vi "Page.Next.vi"(8 "error in (no error)":errorcluster, 11 "State Variables":T1) -> (0 "error out":errorcluster, 3 "State Variables":T1)   [LabVIEW 2015]
uses:
  Types/Main.StateVariables.ctl
  <vilib>/Utility/miscctls.llb/LVPositionTypeDef.ctl
  Types/Execute.UserEventRefs.ctl
  <vilib>/NI Veristand/Execution/Workspace/SystemStateRegEventRef.ctl
  <vilib>/NI Veristand/Execution/Workspace/Target State Info.ctl
  <vilib>/NI Veristand/Execution/Workspace/Target State.ctl
  <vilib>/NI Veristand/Execution/WaveformStreaming/Waveform Data Watcher Event Data (DBL).ctl
  <vilib>/NI Veristand/Execution/WaveformStreaming/WaveformStreamSpecification.ctl
  NationalInstruments.VeriStand.ClientAPI
  <vilib>/NI Veristand/Execution/Workspace/SystemStateEventRef.ctl
  <vilib>/NI Veristand/Execution/Workspace/WorkspaceAPI.ctl
  Types/UI.Object.ctl
  Types/Waveforms.Info.ctl
  <vilib>/NI Veristand/Execution/WaveformStreaming/Registered Waveform Streams Data Event Refnum (DBL).ctl
  <vilib>/NI Veristand/Execution/WaveformStreaming/WaveformDataWatcherDBL.ctl
  <vilib>/NI Veristand/Execution/WaveformStreaming/WaveformStreamingAPI.ctl
  <vilib>/NI Veristand/Execution/Workspace/NI_VS Workspace ExecutionAPI.lvlib
  <vilib>/NI Veristand/Execution/WaveformStreaming/NI_VS Waveform Streaming Interface.lvlib
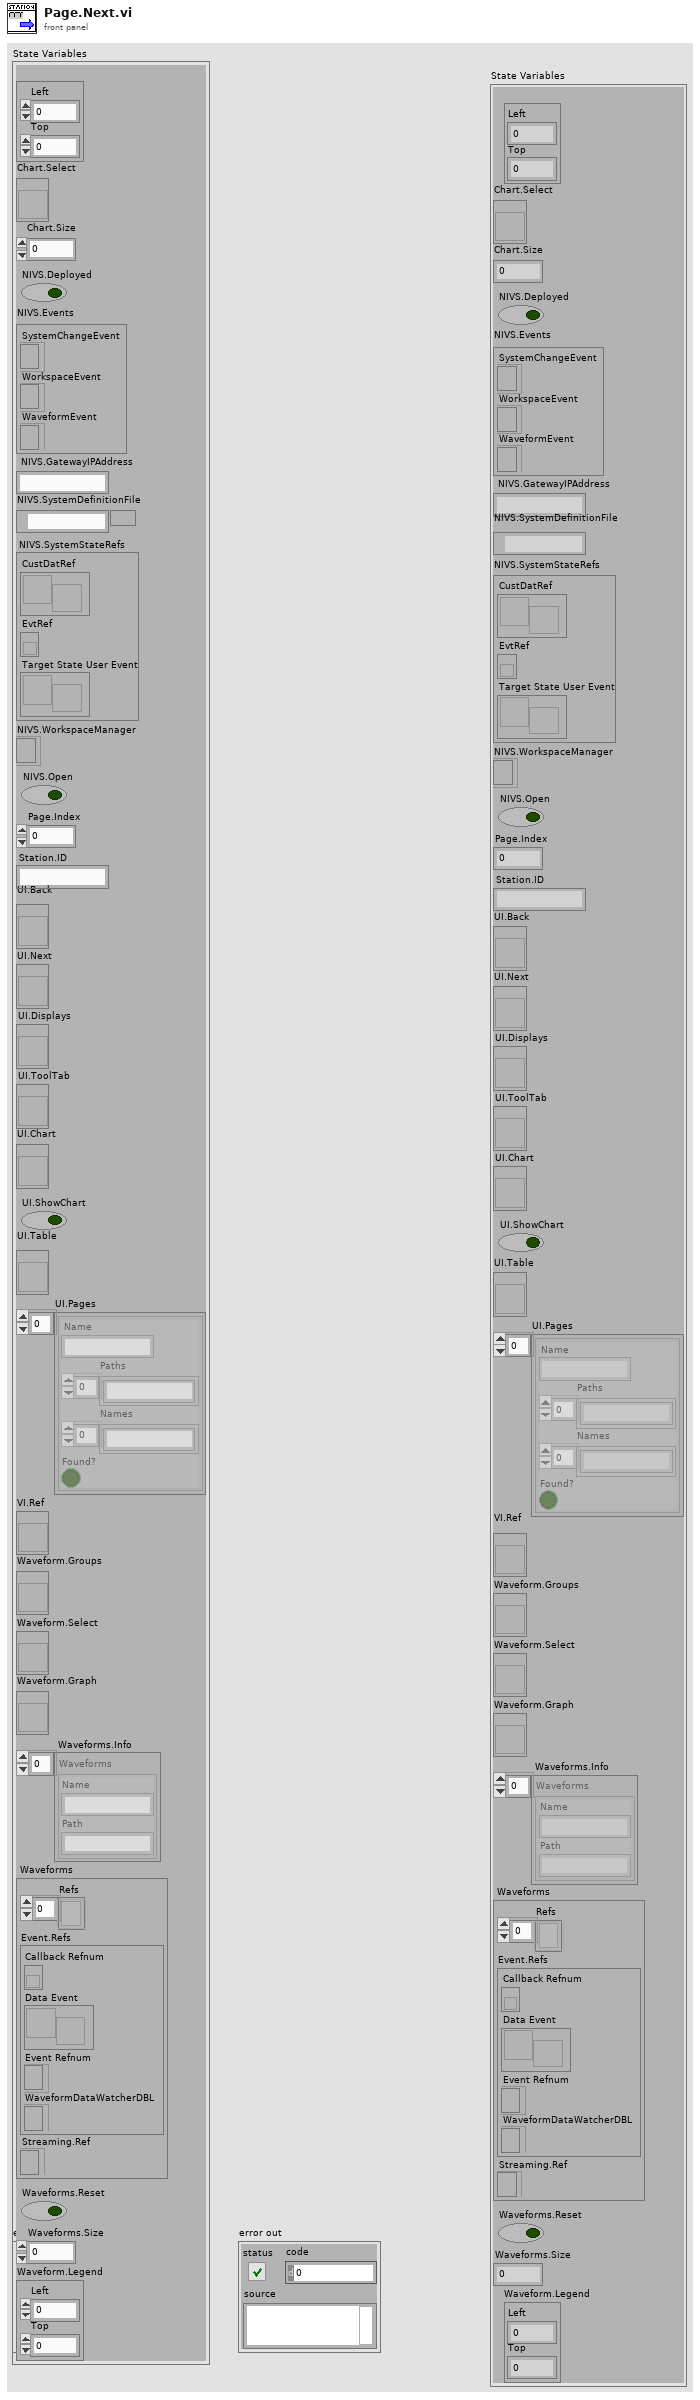
[diagram p1: front panel]
types:
  T1 = typedef "Main.StateVariables.ctl" = cluster{"Chart.Legend":T2, "Chart.Select":refnum<vi>, "Chart.Size":i32, "NIVS.Deployed":bool, "NIVS.Events":T3, "NIVS.GatewayIPAddress":string, "NIVS.SystemDefinitionFile":path, "NIVS.SystemStateRefs":T5, "NIVS.WorkspaceManager":T6, "NIVS.Open":bool, "Page.Index":u32, "Station.ID":string, "UI.Back":refnum<vi>, "UI.Next":refnum<vi>, "UI.Displays":refnum<vi>, "UI.ToolTab":refnum<vi>, "UI.Chart":refnum<vi>, "UI.ShowChart":bool, "UI.Table":refnum<vi>, "UI.Pages":T7[], "VI.Ref":refnum<vi>, "Waveform.Groups":refnum<vi>, "Waveform.Select":refnum<vi>, "Waveform.Graph":refnum<vi>, "Waveforms.Info":T8[], "Waveforms":cluster{"Refs":T9[], "Event.Refs":T10, "Streaming.Ref":T12}, "Waveforms.Reset":bool, "Waveforms.Size":i32, "Waveform.Legend":T2}
  T2 = typedef "LVPositionTypeDef.ctl" = cluster{"Left":i32, "Top":i32}
  T3 = typedef "Execute.UserEventRefs.ctl" = cluster{"SystemChangeEvent":T4, "WorkspaceEvent":refnum<event-registration>, "WaveformEvent":refnum<event-registration>}
  T4 = typedef "NI_VS Workspace ExecutionAPI.lvlib/SystemStateRegEventRef.ctl" = refnum<event-registration>
  T5 = typedef "NI_VS Workspace ExecutionAPI.lvlib/SystemStateEventRef.ctl" = cluster{"CustDatRef":refnum<user-event>, "EvtRef":refnum<k27>, "Target State User Event":refnum<user-event>}
  T6 = typedef "NI_VS Workspace ExecutionAPI.lvlib/WorkspaceAPI.ctl" = refnum<k24>
  T7 = typedef "UI.Object.ctl" = cluster{"Name":string, "Paths":string[], "Names":string[], "Found?":bool}
  T8 = typedef "Waveforms.Info.ctl" = cluster{"Name":string, "Path":string}
  T9 = typedef "NI_VS Waveform Streaming Interface.lvlib/WaveformStreamSpecification.ctl" = refnum<k24>
  T10 = typedef "NI_VS Waveform Streaming Interface.lvlib/Registered Waveform Streams Data Event Refnum (DBL).ctl" = cluster{"Callback Refnum":refnum<k27>, "Data Event":refnum<user-event>, "Event Refnum":refnum<event-registration>, "WaveformDataWatcherDBL":T11}
  T11 = typedef "NI_VS Waveform Streaming Interface.lvlib/WaveformDataWatcherDBL.ctl" = refnum<k24>
  T12 = typedef "NI_VS Waveform Streaming Interface.lvlib/WaveformStreamingAPI.ctl" = refnum<k24>
  T13 = enum8{"Enabled", "Disabled", "Disabled and Grayed Out"}
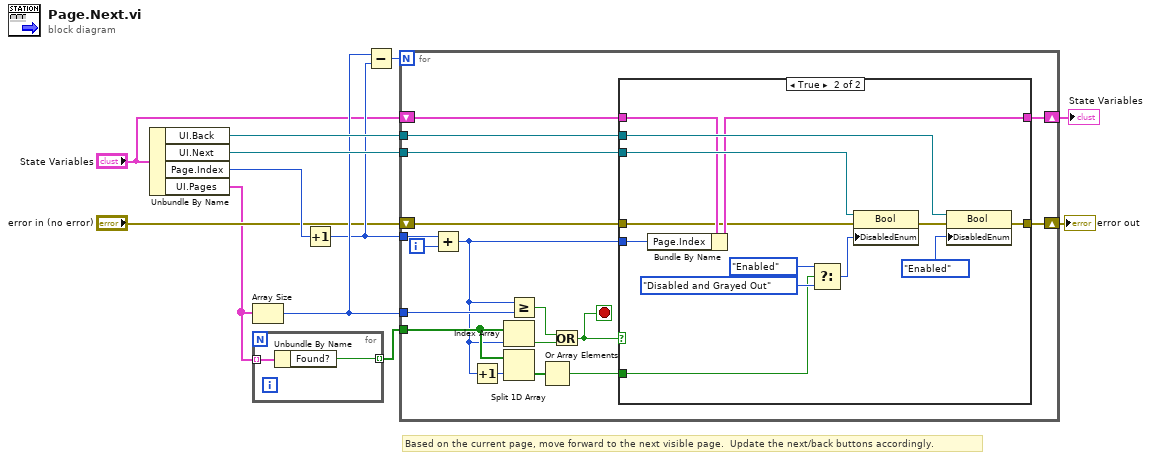
[diagram p0: block diagram]
diagram:
  # "Based on the current page, move forward to the next visible page.  Update the next/back buttons accordingly."
  n1 = Unbundle By Name("State Variables") -> ("UI.Back"=w10:refnum<vi>, "UI.Next"=w11:refnum<vi>, "Page.Index"=w6:u32, "UI.Pages"=w2:T7[])
  n2 = Array Size(array=w2) -> (size(s)=w9:i32)
  n3 = for {
    tunnel: w2 -> [w14] mode=indexing
    tunnel: [w13] -> w1 mode=indexing
    n4 = Unbundle By Name(w14) -> ("Found?"=w13:bool)
  }
  n5 = Increment(x=w6) -> (x+1=w8:u32)
  n6 = Subtract(x=w9, y=w8) -> (x-y=w7:u32)
  n7 = for {
    N: w7 -> [_]
    tunnel: w9 -> [w30]
    tunnel: w8 -> [w22]
    tunnel: w11 -> [w28]
    tunnel: w10 -> [w27]
    shift-right: [w29] -> w12
    shift-left: "error in (no error)" -> [w31]
    tunnel: w1 -> [w23]
    shift-right: [w15] -> w3
    shift-left: "State Variables" -> [w16]
    i -> [w26]
    stop <- w17 stop-if-true
    n8 = Add(x=w22, y=w26) -> (x+y=w21:u32)
    n9 = Increment(x=w21) -> (x+1=w18:u32)
    n10 = Index Array(array=w23, index=w21) -> (element=w24:bool)
    n11 = Split 1D Array(array=w23, index=w18) -> (second subarray=w20:bool[])  [unwired: 1 out]
    n12 = Greater Or Equal?(x=w21, y=w30) -> (x >= y?=w25:bool)
    n13 = Or Array Elements(Boolean array=w20) -> (logical OR=w19:bool)
    n14 = Or(x=w25, y=w24) -> (x .or. y?=w17:bool)
    n15 = case shown="True" w17 {
      tunnel: w31 -> [w33 w34]
      tunnel: [w33 w46] -> w29
      tunnel: w21 -> [_ w36]
      tunnel: w28 -> [_ w40]
      tunnel: w27 -> [_ w39]
      tunnel: w19 -> [_ w38]
      tunnel: w16 -> [w32 w37]
      tunnel: [w32 w35] -> w15
      frame False {
      }
      frame True {
        n16 = Bundle By Name(cluster=w37, "Page.Index"=w36) -> (w35:T1)
        n17 = Select(t=T13."Enabled" ("Disabled"), s=w38, f=T13."Disabled and Grayed Out") -> (s? t:f=w41:T13)
        n18 = property class="Bool"(reference=w40, error in=w34, "DisabledEnum"=w41) -> (error out=w45:errorcluster)  [unwired: 1 out]
        n19 = property class="Bool"(reference=w39, error in=w45, "DisabledEnum"=T13."Enabled" ("Disabled")) -> (error out=w46:errorcluster)  [unwired: 1 out]
      }
    }
  }
  "error out" <- w12
  "State Variables" <- w3
